vi "ReadCurrent.vi"(8 "error in (no error)":errorcluster, 10 "LoopFromMain":bool, 11 "VISA resource name":refnum<visa-resource-name>="COM9") -> (0 "error out":errorcluster, 1 "CurrentSens":bool, 2 "CurrentOut":string)   [LabVIEW 2017]
uses:
  <vilib>/Instr/_visa.llb/VISA Configure Serial Port (Instr).vi
panel:
  out "Delta t":dbl
  out "Array":string[](array[string])
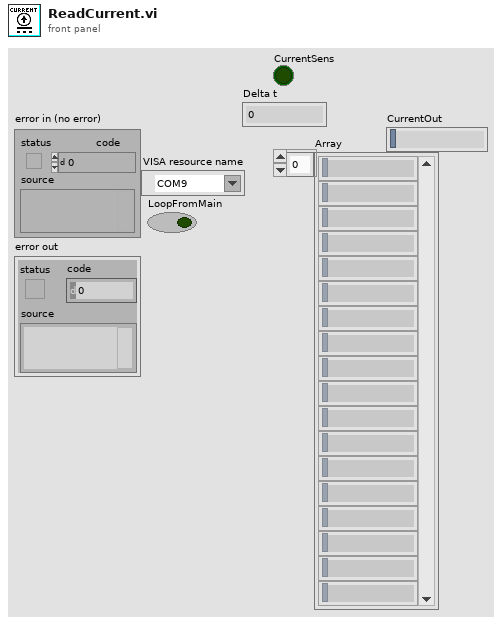
[diagram p1: front panel]
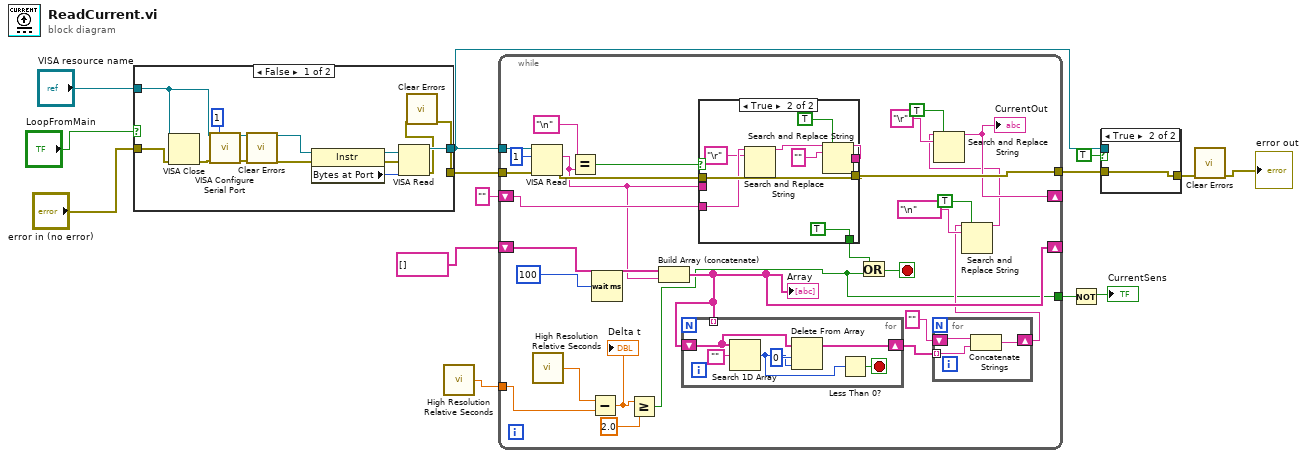
[diagram p0: block diagram]
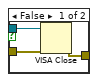
[diagram p2: hidden frame]
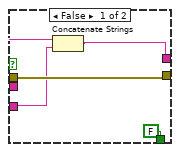
[diagram p4: hidden frame]
diagram:
  n1 = case shown="False" "LoopFromMain" {
    tunnel: [w15 w28] -> w14
    tunnel: "error in (no error)" -> [w20 w28]
    tunnel: "VISA resource name" -> [w18 w29]
    tunnel: [w22 w29] -> w9
    frame False {
      n2 = VISA Close(VISA resource name=w18, error in (no error)=w20) -> (error out=w19:errorcluster)
      n3 = call-poly "VISA Configure Serial Port"("VISA resource name"=w18, "timeout (10sec)"=u32 1, "error in (no error)"=w19) -> ("VISA resource name out"=w17:refnum<visa-resource-name>, "error out"=w24:errorcluster)  [unwired: 11 in]
      n4 = call <vilib>:"Clear Errors.vi"("error in (no error)"=w24) -> ("error out"=w16:errorcluster)  [unwired: 5 in, 1 out]
      n5 = property class="Instr"(reference=w17, error in=w16) -> (reference out=w26:refnum<visa-resource-name>, error out=w25:errorcluster, "Bytes at Port"=w27:u32)
      n6 = VISA Read(VISA resource name=w26, byte count=w27, error in (no error)=w25) -> (VISA resource name out=w22:refnum<visa-resource-name>, error out=w21:errorcluster)  [unwired: 2 out]
      n7 = call <vilib>:"Clear Errors.vi"("error in (no error)"=w21) -> ("error out"=w15:errorcluster)  [unwired: 5 in, 1 out]
    }
    frame True {
    }
  }
  n8 = call <vilib>:"High Resolution Relative Seconds.vi"() -> ("relative seconds"=w4:dbl)
  n9 = while {
    tunnel: w9 -> [w57]
    tunnel: w14 -> [w55]
    tunnel: [w53] -> w8
    shift-right: [w45] -> _
    shift-left: "" -> [w51]
    shift-right: [w42] -> _
    shift-left: string[] [] -> [w47]
    tunnel: w4 -> [w35]
    tunnel: [w30] -> w3
    stop <- w33 stop-if-true
    n10 = VISA Read(VISA resource name=w57, byte count=u32 1, error in (no error)=w55) -> (read buffer=w46:string, error out=w54:errorcluster)  [unwired: 2 out]
    n11 = call <vilib>:"High Resolution Relative Seconds.vi"() -> ("relative seconds"=w34:dbl)
    n12 = Equal?(x="\n", y=w46) -> (x = y?=w48:bool)
    n13 = Subtract(x=w34, y=w35) -> (x-y=w32:dbl)
    "Delta t" <- w32
    n14 = Wait (ms)(milliseconds to wait=u32 100) -> ()  [unwired: 1 out]
    n15 = Greater Or Equal?(x=w32, y=2.0) -> (x >= y?=w30:bool)
    n16 = Build Array (concatenate)(w47, w46) -> (w42:string[])
    "Array" <- w42
    n17 = for {
      tunnel: w42 -> [_] mode=indexing
      shift-right: [w63] -> w41
      shift-left: w42 -> [w64]
      stop <- w62 stop-if-true
      n18 = Search 1D Array(1D array=w64, element="") -> (index of element=w61:i32)  [unwired: 1 in]
      n19 = Delete From Array(array=w64, length=0, index=w61) -> (array with subset deleted=w63:string[])  [unwired: 1 out]
      n20 = Less Than 0?(x=w61) -> (x < 0?=w62:bool)
    }
    n21 = case shown="True" w48 {
      tunnel: [FALSE TRUE] -> w50
      tunnel: w54 -> [w70 w78]
      tunnel: [w70 w78] -> w53
      tunnel: [w67 w72] -> _
      tunnel: w51 -> [w68 w77]
      tunnel: w46 -> [w69 _]
      frame False {
        n22 = Concatenate Strings(w69, w68) -> (w67:string)
      }
      frame True {
        n23 = Search and Replace String(input string=w77, search string="\r") -> (result string=w75:string)  [unwired: 6 in, 3 out]
        n24 = Search and Replace String(replace all?=TRUE ("replace all? (F)"), input string=w75, search string="") -> (result string=w72:string)  [unwired: 5 in, 3 out]
      }
    }
    n25 = Or(x=w50, y=w30) -> (x .or. y?=w33:bool)
    n26 = for {
      tunnel: w41 -> [w58] mode=indexing
      shift-right: [w60] -> w37
      shift-left: "" -> [w59]
      n27 = Concatenate Strings(w59, w58) -> (w60:string)
    }
    n28 = Search and Replace String(replace all?=TRUE ("replace all? (F)"), input string=w37, search string="\n") -> (result string=w36:string)  [unwired: 5 in, 3 out]
    n29 = Search and Replace String(replace all?=TRUE ("replace all? (F)"), input string=w36, search string="\r") -> (result string=w45:string)  [unwired: 5 in, 3 out]
    "CurrentOut" <- w45
  }
  n30 = Not(x=w3) -> (.not. x?=→"CurrentSens":bool)
  n31 = case shown="True" TRUE {
    tunnel: w9 -> [w82 _]
    tunnel: w8 -> [w81 w83]
    tunnel: [w80 w83] -> w7
    frame False {
      n32 = VISA Close(VISA resource name=w82, error in (no error)=w81) -> (error out=w80:errorcluster)
    }
    frame True {
    }
  }
  n33 = call <vilib>:"Clear Errors.vi"("error in (no error)"=w7) -> ("error out"=→"error out":errorcluster)  [unwired: 5 in, 1 out]
